vi "Run Instrument.vi"(8 "error in":errorcluster, 11 "Open Path CRD in":refnum<class "Open Path CRD.lvclass">) -> (0 "error out":errorcluster)   [LabVIEW 2015]
doc: "This is the main OPCRD instrument interface."
uses:
  CRD/Open Path CRD.lvclass
  Reusable/Instrument/state.ctl
  Reusable/Session Log/System Log.lvclass
  Reusable/Session Log/System Log.lvclass/System Log.ctl
  Reusable/Instrument/Instrument.lvclass/Instrument.ctl
  Reusable/Session Log/Accessors/Write Main Path.vi
  Reusable/Instrument/Write Log Session.vi
  Reusable/Instrument/Instrument.lvclass
  <userlib>/_Session Fwk/Session - Root.lvclass
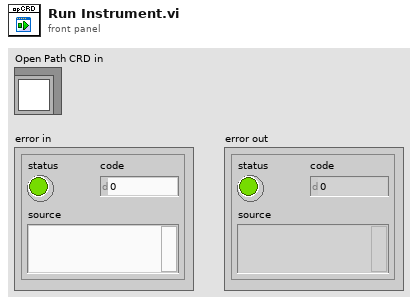
[diagram p1: front panel]
types:
  T1 = typedef "Instrument.lvclass/state.ctl" = enum8{"Configure", "Acquire", "Wait", "Quit", "Handle Error", "NOOP"}
  T2 = typedef "Session - Root.lvclass/Session Handle.ctl" = refnum<data-value>
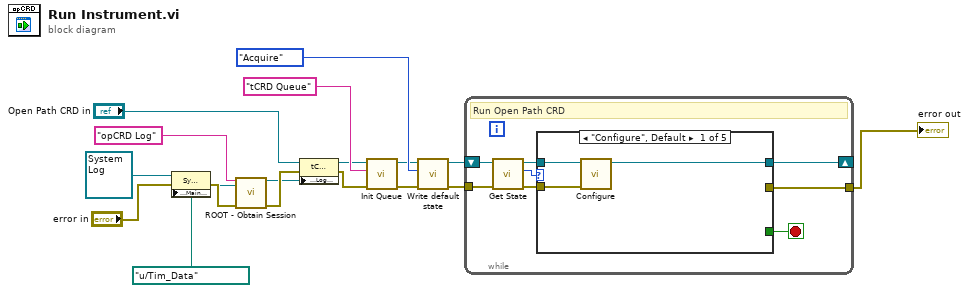
[diagram p0: block diagram]
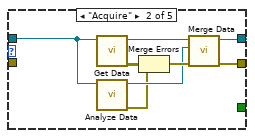
[diagram p2: hidden frame]
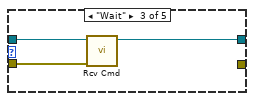
[diagram p3: hidden frame]
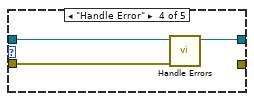
[diagram p4: hidden frame]
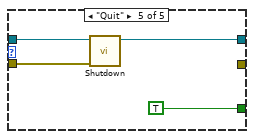
[diagram p5: hidden frame]
diagram:
  n1 = property class="Sys Log"(reference=refnum<class "System Log.lvclass"> refnum ("Sys Log"), error in="error in", "Accessors:Main Path"=path "u:/Tim_Data" ("RD Data Path")) -> (reference out=w10:refnum<class "System Log.lvclass">, error out=w11:errorcluster)
  n2 = call <userlib>:"ROOT - Obtain Session.vi"("Session Name ()"="opCRD Log", "OBJ - Session"=w10, "error in (no error)"=w11) -> ("Session Handle"=w13:T2, "error out"=w14:errorcluster)  [unwired: 10 in, 1 out]
  n3 = property class="tCRD"(reference="Open Path CRD in", error in=w14, "Accessors:Log Session"=w13) -> (reference out=w1:refnum<class "Open Path CRD.lvclass">, error out=w15:errorcluster)
  n4 = call "Init Queue.vi"("error in"=w15, "queue_name"="tCRD Queue", "Instrument in"=w1) -> ("error out"=w3:errorcluster, "Instrument out"=w4:refnum<class "Open Path CRD.lvclass">)  [unwired: 7 in]
  n5 = call "Write default state.vi"("error in (no error)"=w3, "instr state"=state."Acquire", "Instrument in"=w4) -> ("error out"=w17:errorcluster, "Instrument out"=w5:refnum<class "Open Path CRD.lvclass">)  [unwired: 7 in]
  n6 = while "Acquisition" {
    tunnel: w17 -> [w26]
    shift-right: [w23] -> _
    shift-left: w5 -> [w25]
    tunnel: [w22] -> w18
    stop <- w24 stop-if-true
    # "Run Open Path CRD"
    n7 = call "Get State.vi"("error in"=w26, "Instrument in"=w25) -> ("error out"=w19:errorcluster, "default state"=w21:T1, "Instrument out"=w20:refnum<class "Open Path CRD.lvclass">)  [unwired: 7 in]
    n8 = case shown="\"Configure\", Default" w21 {
      tunnel: w20 -> [w29 w36 w39 w43 w46]
      tunnel: w19 -> [w28 _ w38 w42 w45]
      tunnel: [_ _ _ _ TRUE] -> w24
      tunnel: [w27 w37 w40 w41 w44] -> w23
      tunnel: [_ w35 _ _ _] -> w22
      frame "Configure", Default {
        n9 = call-dynamic "Configure.vi"("error in"=w28, "tCRD in"=w29) -> ("tCRD out"=w27:refnum<class "Open Path CRD.lvclass">)  [unwired: 8 in, 1 out]
      }
      frame "Acquire" {
        n10 = call-dynamic "Get Data.vi"("tCRD in"=w36) -> ("error out"=w31:errorcluster, "tCRD out"=w34:refnum<class "Open Path CRD.lvclass">)  [unwired: 9 in]
        n11 = call-dynamic "Analyze Data.vi"("tCRD in"=w36) -> ("error out"=w30:errorcluster, "tCRD out"=w32:refnum<class "Open Path CRD.lvclass">)  [unwired: 9 in]
        n12 = Merge Errors(w31, w30) -> (w33:errorcluster)
        n13 = call-dynamic "Merge Data.vi"("error in"=w33, "Analyzed"=w32, "Acquired"=w34) -> ("error out"=w35:errorcluster, "tCRD out"=w37:refnum<class "Open Path CRD.lvclass">)  [unwired: 7 in]
      }
      frame "Wait" {
        n14 = call-dynamic "Rcv Cmd.vi"("error in"=w38, "tCRD in"=w39) -> ("tCRD out"=w40:refnum<class "Open Path CRD.lvclass">)  [unwired: 8 in, 1 out]
      }
      frame "Handle Error" {
        n15 = call-dynamic "Handle Errors.vi"("error in"=w42, "tCRD in"=w43) -> ("tCRD out"=w41:refnum<class "Open Path CRD.lvclass">)  [unwired: 7 in, 2 out]
      }
      frame "Quit" {
        n16 = call-dynamic "Shutdown.vi"("error in"=w45, "tCRD in"=w46) -> ("tCRD out"=w44:refnum<class "Open Path CRD.lvclass">)  [unwired: 8 in, 1 out]
      }
    }
  }
  "error out" <- w18
